vi "Node - Connect.vi"(8 "error in (no error)":errorcluster, 10 "Configuration Properties In":T3, 11 "Node Data In":T1) -> (0 "error out":errorcluster, 2 "Configuration Properties Out":T3, 3 "Node Data Out":T1)   [LabVIEW 2016, in "PXImc Custom Device Engine.lvlib" / "PXImc Router.lvlib"]
uses:
  PXImc Router.lvlib
  Controls/Node Data.ctl
  Controls/Table Index-Size.ctl
  Controls/Node - Configuration.ctl
  <vilib>/pximc/Connect (DBL).vi
  <vilib>/pximc/nipximc.lvlib
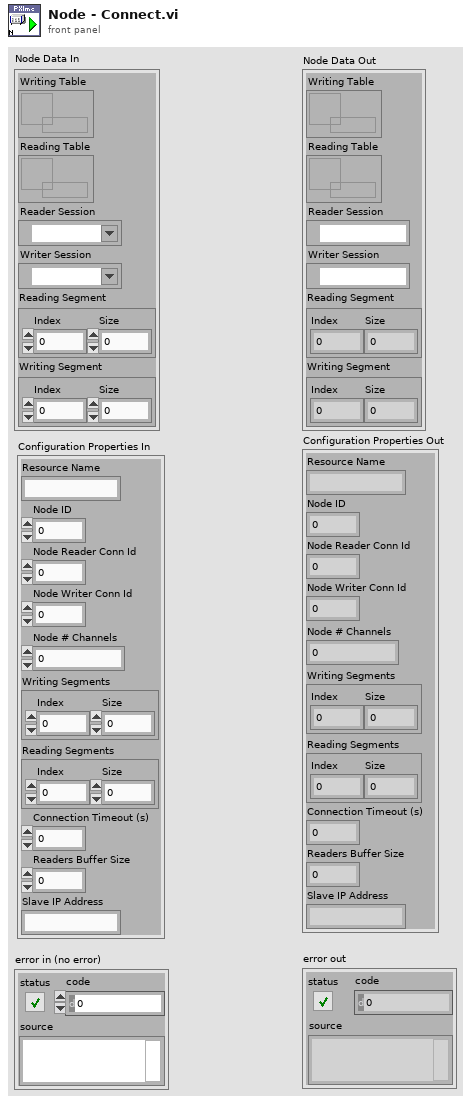
[diagram p1: front panel]
types:
  T1 = typedef "PXImc Custom Device Engine.lvlib/PXImc Router.lvlib/Node Data.ctl" = cluster{"Writing Table":refnum<data-value>, "Reading Table":refnum<data-value>, "Reader Session":refnum<k21>, "Writer Session":refnum<k21>, "Reading Segment":T2, "Writing Segment":T2}
  T2 = typedef "PXImc Custom Device Engine.lvlib/PXImc Router.lvlib/Table Index-Size.ctl" = cluster{"Index":u32, "Size":u32}
  T3 = typedef "PXImc Custom Device Engine.lvlib/PXImc Router.lvlib/Node - Configuration.ctl" = cluster{"Resource Name":string, "Node ID":u16, "Node Reader Conn Id":u16, "Node Writer Conn Id":u16, "Node # Channels":u32, "Writing Segments":T2, "Reading Segments":T2, "Connection Timeout (s)":dbl, "Readers Buffer Size":u32, "Slave IP Address":string}
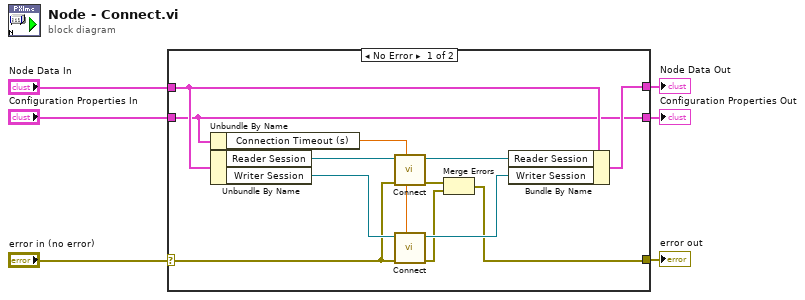
[diagram p0: block diagram]
diagram:
  n1 = case shown="No Error" "error in (no error)" {
    selector: "error in (no error)" -> [w10 w19]
    tunnel: "Configuration Properties In" -> [w11 w20]
    tunnel: "Node Data In" -> [w14 w21]
    tunnel: [w12 w21] -> w3
    tunnel: [w11 w20] -> w4
    tunnel: [w7 w19] -> w1
    frame No Error {
      n2 = Unbundle By Name(w11) -> ("Connection Timeout (s)"=w17:dbl)
      n3 = Unbundle By Name(w14) -> ("Reader Session"=w13:refnum<k21>, "Writer Session"=w18:refnum<k21>)
      n4 = call-poly <vilib>:"Connect.vi"("timeout in seconds (-1)"=w17, "error in (no error)"=w10, "session in"=w13) -> ("error out"=w9:errorcluster, "session out"=w16:refnum<k21>)  [unwired: 7 in]
      n5 = call-poly <vilib>:"Connect.vi"("timeout in seconds (-1)"=w17, "error in (no error)"=w10, "session in"=w18) -> ("error out"=w8:errorcluster, "session out"=w15:refnum<k21>)  [unwired: 7 in]
      n6 = Merge Errors(w9, w8) -> (w7:errorcluster)
      n7 = Bundle By Name(cluster=w14, "Reader Session"=w16, "Writer Session"=w15) -> (w12:T1)
    }
    frame Error {
    }
  }
  "Configuration Properties Out" <- w4
  "Node Data Out" <- w3
  "error out" <- w1
